vi "Run.vi"(0 "Joystick ID":refnum<k1>, 2 "Joystick event":T4, 4 "Stop event":refnum<user-event>, 5 "error in":errorcluster) -> (14 "Joystick ID out":refnum<k1>, 19 "error out":errorcluster)   [LabVIEW 2018]
uses:
  Joystick event.ctl
  <vilib>/Utility/inputDevices.llb/joystickAcquire.vi
panel:
  out "direction info":T1
  out "axis info":T2
  out "cluster":T3
  out "Joystick buttons":bool[](array[boolean])
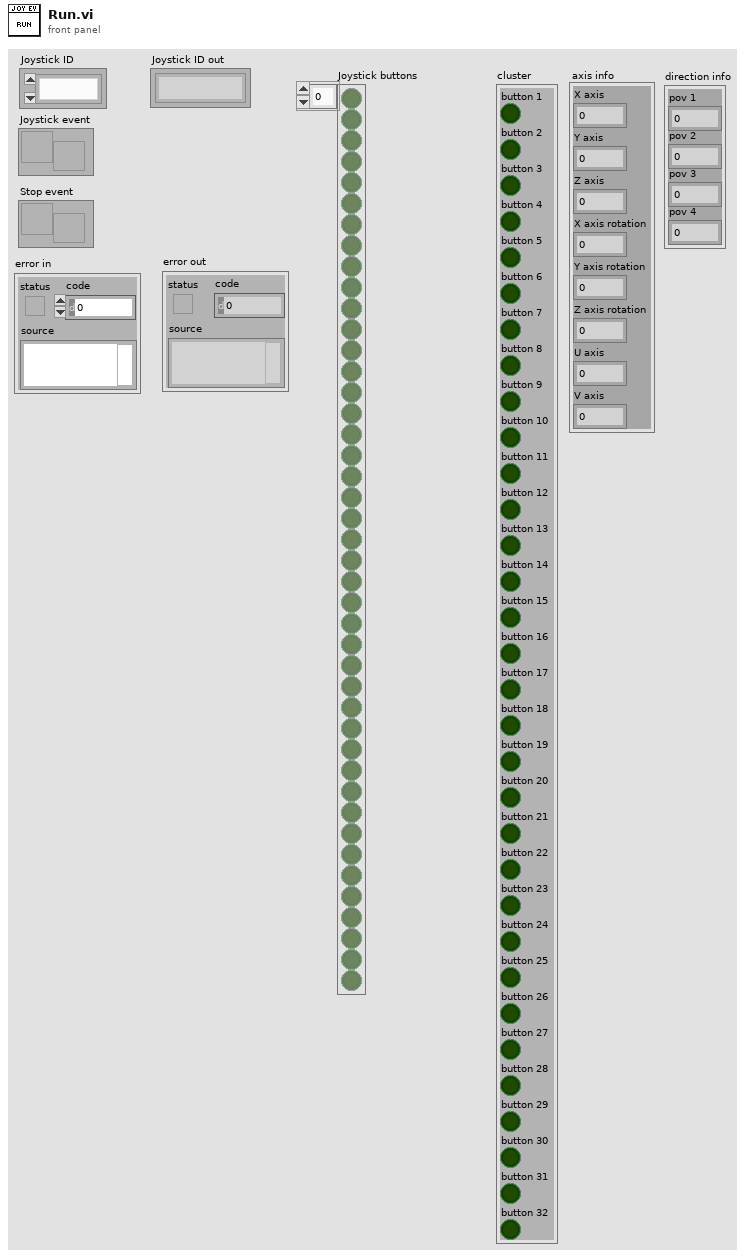
[diagram p1: front panel]
types:
  T1 = cluster{"pov 1":i32, "pov 2":i32, "pov 3":i32, "pov 4":i32}
  T2 = cluster{"X axis":i32, "Y axis":i32, "Z axis":i32, "X axis rotation":i32, "Y axis rotation":i32, "Z axis rotation":i32, "U axis":i32, "V axis":i32}
  T3 = cluster{"button 1":bool, "button 2":bool, "button 3":bool, "button 4":bool, "button 5":bool, "button 6":bool, "button 7":bool, "button 8":bool, "button 9":bool, "button 10":bool, "button 11":bool, "button 12":bool, "button 13":bool, "button 14":bool, "button 15":bool, "button 16":bool, "button 17":bool, "button 18":bool, "button 19":bool, "button 20":bool, "button 21":bool, "button 22":bool, "button 23":bool, "button 24":bool, "button 25":bool, "button 26":bool, "button 27":bool, "button 28":bool, "button 29":bool, "button 30":bool, "button 31":bool, "button 32":bool}
  T4 = typedef "Joystick event.ctl" = refnum<user-event>
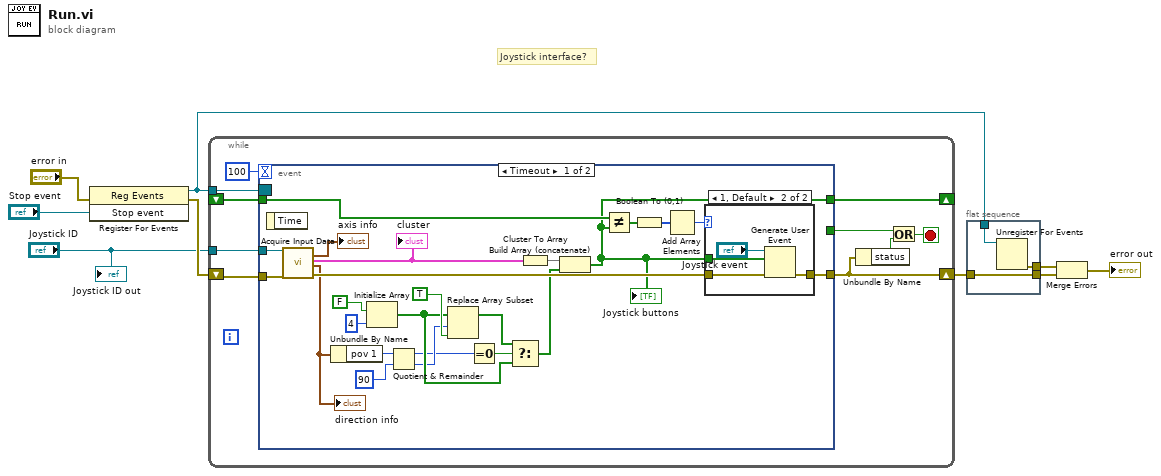
[diagram p0: block diagram]
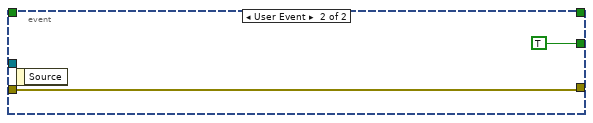
[diagram p3: hidden frame]
diagram:
  # "Joystick interface?"
  n1 = register-events(error in="error in", "Stop event") -> (reference out=w7:refnum<event-registration>, error out=w8:errorcluster)  [unwired: 1 in]
  n2 = while {
    tunnel: "Joystick ID" -> [w18]
    shift-right: [w13] -> w2
    shift-left: w8 -> [w19]
    shift-right: [w16] -> _
    shift-left: _ -> [w15]
    tunnel: w7 -> [w14]
    stop <- w10 stop-if-true
    n3 = event shown="[0] Timeout" {
      selector: w14 -> [_ _]
      dyn-events: _ -> [_ _]
      timeout: 100 -> [_ _]
      tunnel: w19 -> [w43 w49]
      tunnel: w18 -> [w42 _]
      tunnel: [w40 w49] -> w13
      tunnel: [_ TRUE] -> w11
      tunnel: [w26 _] -> w16
      tunnel: w15 -> [w37 _]
      event Timeout {
        n4 = event-data() -> ()  [unwired: 1 in, 1 out]
        n5 = call-poly <vilib>:"Acquire Input Data.vi"("device ID"=w42, "error in (no error)"=w43) -> ("axis info"=→"axis info":T2, "button info"=w35:T3, "direction info"=w33:T1, "error out"=w41:errorcluster)  [unwired: 13 in, 1 out]
        "cluster" <- w35
        "direction info" <- w33
        n6 = Unbundle By Name(w33) -> ("pov 1"=w31:i32)
        n7 = Initialize Array(FALSE ("button 1"), 4 ("dimension size")) -> (w22:bool[])
        n8 = Quotient & Remainder(x=w31, y=90) -> (x-y*floor(x/y)=w20:i32, floor(x/y)=w21:i32)
        n9 = Replace Array Subset(array=w22, new element=TRUE ("new element/subarray"), index=w21) -> (w28:bool[])
        n10 = Equal To 0?(x=w20) -> (x = 0?=w29:bool)
        n11 = Select(t=w28, s=w29, f=w22) -> (s? t:f=w25:bool[])
        n12 = Cluster To Array(cluster=w35) -> (array=w27:bool[])
        n13 = Build Array (concatenate)(w27, w25) -> (w26:bool[])
        "Joystick buttons" <- w26
        n14 = Not Equal?(x=w37, y=w26) -> (x != y?=w36:bool[])
        n15 = Boolean To (0,1)(Boolean=w36) -> (0, 1=w39:i16[])
        n16 = Add Array Elements(numeric array=w39) -> (sum=w38:i16)
        n17 = case shown="1, Default" w38 {
          tunnel: w41 -> [w44 w47]
          tunnel: [w44 w46] -> w40
          tunnel: w26 -> [_ w45]
          frame 0 {
          }
          frame 1, Default {
            n18 = Generate User Event(user event="Joystick event", event data cluster=w45, error in=w47) -> (error out=w46:errorcluster)  [unwired: 1 in, 1 out]
          }
        }
      }
      event User Event {
        n19 = event-data() -> ()  [unwired: 1 in, 1 out]
      }
    }
    n20 = Unbundle By Name(w13) -> ("status"=w12:bool)
    n21 = Or(x=w11, y=w12) -> (x .or. y?=w10:bool)
  }
  n22 = flat-sequence {
    tunnel: w7 -> [w53]
    tunnel: [w52] -> w4
    tunnel: w2 -> [w51]
    tunnel: [w51] -> w1
    frame #0 {
      n23 = Unregister For Events(event registration refnum=w53) -> (error out=w52:errorcluster)  [unwired: 1 in]
    }
  }
  n24 = Merge Errors(w4, w1) -> (→"error out":errorcluster)
  "Joystick ID out" <- "Joystick ID"
